vi "DriveNetwork.vi"(8 "error in (no error)":errorcluster) -> (0 "error out":errorcluster)   [LabVIEW 2023]
doc: "Network for Drive\n\nInputs:\n -- Error in -- Error cluster -- propagated error input\n\nOutputs:\n -- Error out -- Error cluster -- progated error output"
uses:
  DriveGlobal.vi
  <vilib>/Rock Robotics/Network Tables/NT Write Number.vi
  <vilib>/Rock Robotics/Network Tables/NT Write Boolean.vi
  <vilib>/Rock Robotics/Network Tables/NT Read Number.vi
  <vilib>/Rock Robotics/Network Tables/NT Read Boolean.vi
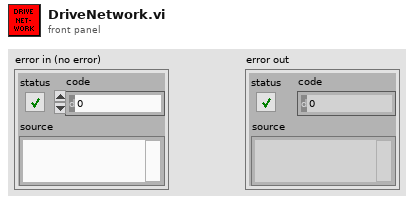
[diagram p1: front panel]
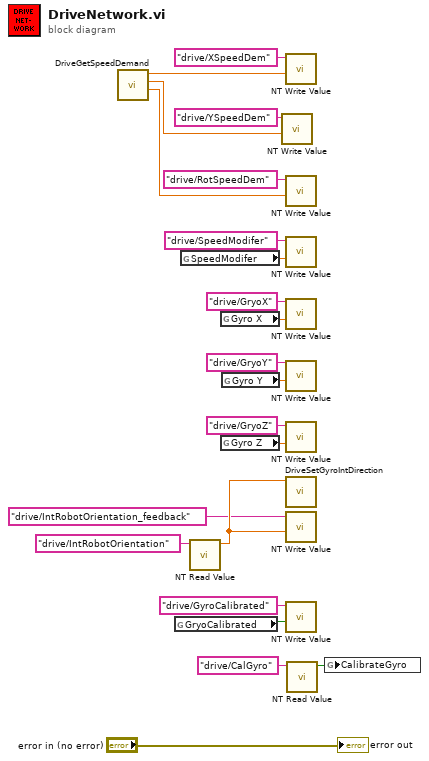
[diagram p0: block diagram]
diagram:
  n1 = call "DriveGetSpeedDemand.vi"() -> ("vOmega"=w4:dbl, "vY"=w20:dbl, "vX"=w21:dbl)  [unwired: 8 in, 1 out]
  n2 = global read "DriveGlobal.vi" "GryoCalibrated"() -> (w6:bool)
  n3 = global read "DriveGlobal.vi" "SpeedModifer"() -> (w12:dbl)
  n4 = call-poly <vilib>:"NT Read Value.vi"("name"="drive/IntRobotOrientation") -> ("value"=w2:dbl)  [unwired: 8 in, 2 out]
  n5 = global read "DriveGlobal.vi" "Gyro X"() -> (w14:dbl)
  n6 = global read "DriveGlobal.vi" "Gyro Z"() -> (w16:dbl)
  n7 = global read "DriveGlobal.vi" "Gyro Y"() -> (w15:dbl)
  n8 = call-poly <vilib>:"NT Write Value.vi"("value"=w20, "name"="drive/YSpeedDem") -> ()  [unwired: 9 in, 1 out]
  n9 = call-poly <vilib>:"NT Write Value.vi"("value"=w21, "name"="drive/XSpeedDem") -> ()  [unwired: 9 in, 1 out]
  n10 = call-poly <vilib>:"NT Write Value.vi"("value"=w4, "name"="drive/RotSpeedDem") -> ()  [unwired: 9 in, 1 out]
  n11 = call-poly <vilib>:"NT Write Value.vi"("value"=w12, "name"="drive/SpeedModifer") -> ()  [unwired: 9 in, 1 out]
  n12 = call-poly <vilib>:"NT Write Value.vi"("value"=w14, "name"="drive/GryoX") -> ()  [unwired: 9 in, 1 out]
  n13 = call-poly <vilib>:"NT Write Value.vi"("value"=w15, "name"="drive/GryoY") -> ()  [unwired: 9 in, 1 out]
  n14 = call-poly <vilib>:"NT Write Value.vi"("value"=w16, "name"="drive/GryoZ") -> ()  [unwired: 9 in, 1 out]
  n15 = call "DriveSetGyroIntDirection.vi"("GyroIntDirection"=w2) -> ()  [unwired: 11 in]
  n16 = call-poly <vilib>:"NT Write Value.vi"("value"=w2, "name"="drive/IntRobotOrientation_feedback") -> ()  [unwired: 9 in, 1 out]
  n17 = call-poly <vilib>:"NT Write Value.vi"("value"=w6, "name"="drive/GyroCalibrated") -> ()  [unwired: 9 in, 1 out]
  n18 = call-poly <vilib>:"NT Read Value.vi"("name"="drive/CalGyro") -> ("value"=w7:bool)  [unwired: 8 in, 2 out]
  n19 = global write "DriveGlobal.vi" "CalibrateGyro"(w7) -> ()
  "error out" <- "error in (no error)"
